vi "discover channels.vi"(8 "error in":errorcluster, 10 "component configuration":refnum<class "TBM module configuration.lvclass">, 11 "asynchronous execution module runtime In":refnum<class "asynchronous execution module runtime.lvclass">) -> (0 "error out":errorcluster, 2 "updated configuration":refnum<class "TBM module configuration.lvclass">, 3 "asynchronous execution module runtime Out":refnum<class "asynchronous execution module runtime.lvclass">)   [LabVIEW 2013, in "asynchronous execution module runtime.lvclass"]
doc: "Provides an interface for discovering channels at runtime. While this interface performs no operations, a child should provide an override which performs discovery of any channel information that may be available at run time and not at configure time."
uses:
  asynchronous execution module runtime.lvclass
  <vilib>/NI/Tag Bus Module Framework/module configuration/TBM module configuration.lvclass
  configuration/asynchronous execution module configuration.lvclass
  asynchronous execution module runtime.lvclass/asynchronous execution module runtime.ctl
  <vilib>/NI/Tag Bus Module Framework/runtime/TBM module execution interface.lvclass
  configuration/asynchronous execution module configuration.lvclass/asynchronous execution module configuration.ctl
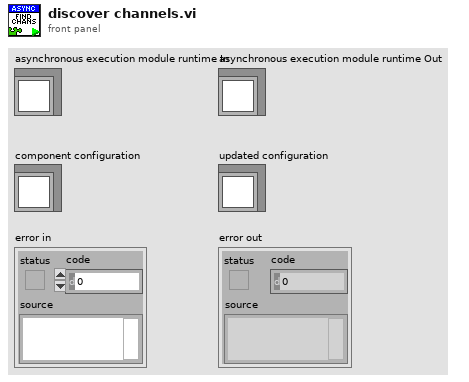
[diagram p1: front panel]
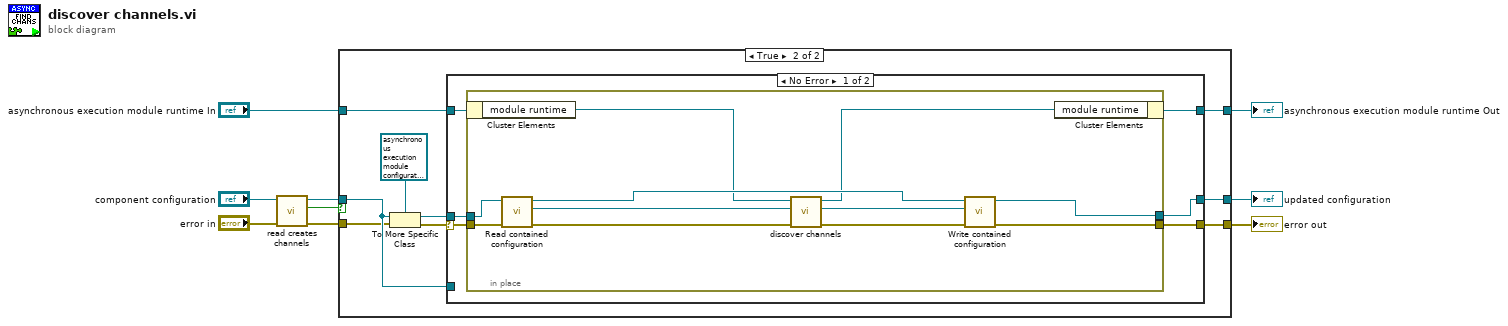
[diagram p0: block diagram]
diagram:
  n1 = call-dynamic "read creates channels.vi"("error in"="error in", "module configuration in"="component configuration") -> ("error out"=w4:errorcluster, "creates channels?"=w2:bool, "module configuration out"=w6:refnum<class "TBM module configuration.lvclass">)  [unwired: 7 in]
  n2 = case shown="True" w2 {
    tunnel: "asynchronous execution module runtime In" -> [w11 w18]
    tunnel: [w11 w17] -> w8
    tunnel: [w10 w16] -> w7
    tunnel: w6 -> [w12 w15]
    tunnel: w4 -> [w10 w14]
    tunnel: [w12 w13] -> w1
    frame False {
    }
    frame True {
      n3 = To More Specific Class(target class=refnum<class "asynchronous execution module configuration.lvclass"> refnum ("CVT Access Configuration"), reference=w15, error in=w14) -> (specific class reference=w19:refnum<class "asynchronous execution module configuration.lvclass">, error out=w20:errorcluster)
      n4 = case shown="No Error" w20 {
        selector: w20 -> [w27 w40]
        tunnel: w19 -> [w25 _]
        tunnel: w18 -> [w26 w41]
        tunnel: [w24 w41] -> w17
        tunnel: [w23 w40] -> w16
        tunnel: w15 -> [_ w39]
        tunnel: [w22 w39] -> w13
        frame No Error {
          n5 = in-place {
            in-place-border: w27 -> [w30]
            in-place-border: w25 -> [w38]
            in-place-border: [w36] -> w23
            in-place-border: [w35] -> w22
            n6 = in-place-cluster #1(w26) -> ("module runtime"=w34:refnum<class "TBM module execution interface.lvclass">)
            n7 = call "Read contained configuration.vi"("error in"=w30, "asynchronous execution module configuration in"=w38) -> ("error out"=w29:errorcluster, "module configuration"=w28:refnum<class "TBM module configuration.lvclass">, "asynchronous execution module configuration out"=w37:refnum<class "asynchronous execution module configuration.lvclass">)  [unwired: 7 in]
            n8 = call-dynamic "discover channels.vi"("error in"=w29, "module configuration"=w28, "module in"=w34) -> ("error out"=w32:errorcluster, "updated configuration"=w31:refnum<class "TBM module configuration.lvclass">, "module out"=w33:refnum<class "TBM module execution interface.lvclass">)  [unwired: 6 in]
            n9 = call "Write contained configuration.vi"("error in"=w32, "module configuration"=w31, "asynchronous execution module configuration in"=w37) -> ("error out"=w36:errorcluster, "asynchronous execution module configuration out"=w35:refnum<class "asynchronous execution module configuration.lvclass">)  [unwired: 7 in]
            n10 = in-place-cluster #1("module runtime"=w33) -> (w24:refnum<class "asynchronous execution module runtime.lvclass">)
          }
        }
        frame Error {
        }
      }
    }
  }
  "error out" <- w7
  "asynchronous execution module runtime Out" <- w8
  "updated configuration" <- w1
